vi "PM100D_Read.vi"(3 "error in (no error)":errorcluster, 4 "Command":string, 6 "VISA in":refnum<visa-resource-name>="COM1") -> (0 "error out":errorcluster, 1 "ReadValue":string, 2 "VISA out":refnum<visa-resource-name>)   [LabVIEW 2014]
doc: "Reads data from the connected instrument. All query commands according the SCPI command table are terminated by a question mark (?)"
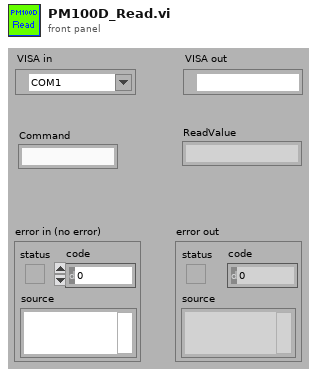
[diagram p1: front panel]
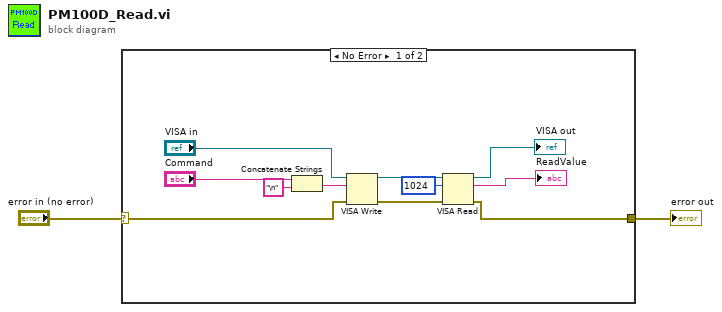
[diagram p0: block diagram]
diagram:
  n1 = case shown="No Error" "error in (no error)" {
    selector: "error in (no error)" -> [w3 w14]
    tunnel: [w4 w14] -> w2
    frame No Error {
      n2 = Concatenate Strings("Command", "\n" ("String")) -> (w11:string)
      n3 = VISA Write(VISA resource name="VISA in", write buffer=w11, error in (no error)=w3) -> (VISA resource name out=w9:refnum<visa-resource-name>, error out=w6:errorcluster)  [unwired: 1 out]
      n4 = VISA Read(VISA resource name=w9, byte count=u32 1024, error in (no error)=w6) -> (VISA resource name out=→"VISA out":refnum<visa-resource-name>, read buffer=→"ReadValue":string, error out=w4:errorcluster)  [unwired: 1 out]
    }
    frame Error {
    }
  }
  "error out" <- w2
